vi "FutekLoadCell.vi"(1 "Futek Sensor Reading":dbl) -> (0 "Futek Force":dbl)   [LabVIEW 2020]
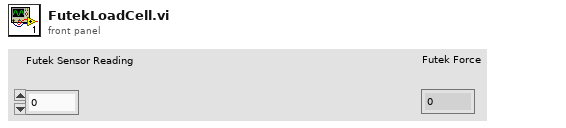
[diagram p1: front panel]
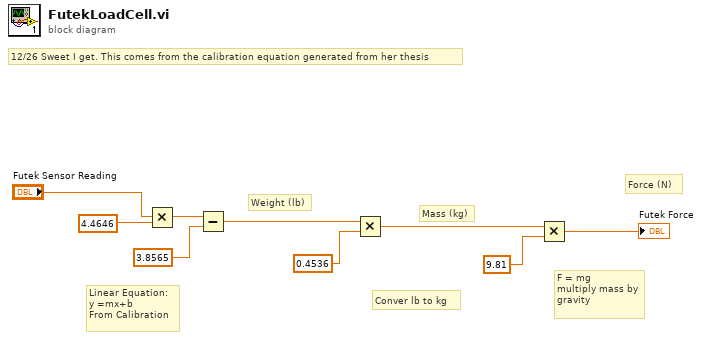
[diagram p0: block diagram]
diagram:
  # "12/26 Sweet I get. This comes from the calibration equation generated from her thesis"
  # "Mass (kg)"
  # "F = mg\nmultiply mass by gravity"
  # "Force (N)"
  # "Conver lb to kg"
  # "Weight (lb)"
  # "Linear Equation:\ny =mx+b\nFrom Calibration"
  n1 = Multiply(x="Futek Sensor Reading", y=4.4646 ("x")) -> (x*y=w8:dbl)
  n2 = Subtract(x=w8, y=3.8565 ("x")) -> (x-y=w6:dbl)
  n3 = Multiply(x=w6, y=0.4536) -> (x*y=w4:dbl)
  n4 = Multiply(x=w4, y=9.81) -> (x*y=→"Futek Force":dbl)
